vi "fpga_RefCounter.vi"(7 "reset":bool, 9 "input valid?":bool, 10 "Reference index":u8, 11 "NChan":u8) -> (1 "Reference channel input valid":bool, 3 "Multichannel enable":bool)   [LabVIEW 2011, in "NI_EP_Resample_FPGA.lvlib"]
uses:
  <vilib>/rvi/FXPMathLib/basic elements/FxpAddSub/XNode/nifxpmath_AddSub.xnode
  <vilib>/addons/Electrical Power/PQ/Resampling/NI_EP_Resample_FPGA.lvlib
  <vilib>/rvi/FXPMathLib/sim/FxpSim.dll
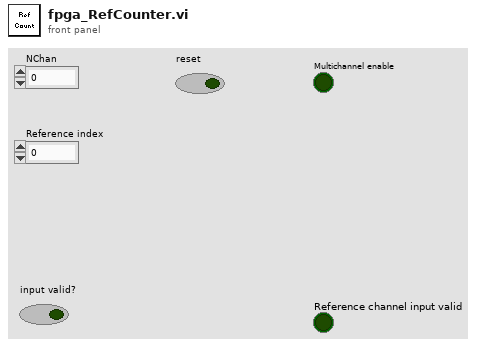
[diagram p1: front panel]
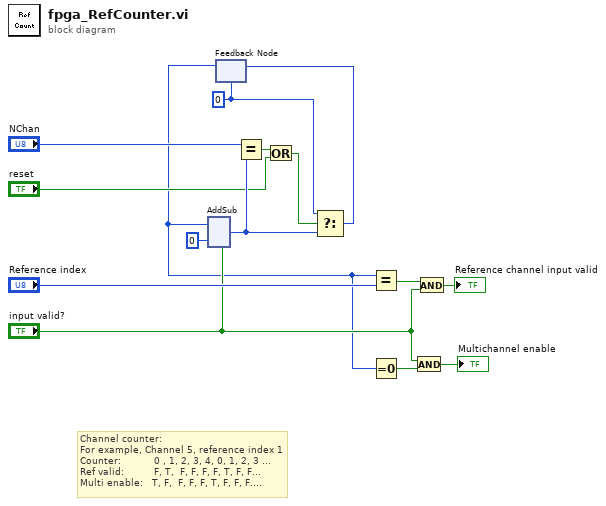
[diagram p0: block diagram]
diagram:
  w9 = u8 0 ("s")
  # "Channel counter:\nFor example, Channel 5, reference index 1\nCounter:           0 , 1, 2, 3, 4, 0, 1, 2, 3 ...\nRef valid:          F, T,  F, F, F, F, T, F, F...\nMulti enable:   T, F,  F, F, F, T, F, F, F...."
  n1 = feedback #1(w9) -> (w1:u8)
  n2 = xnode "AddSub"("x"=w1, "y"=u8 0, "carry-in"="input valid?") -> ("s"=w5:u8)  [unwired: 1 out]
  n3 = Equal?(x="NChan", y=w5) -> (x = y?=w4:bool)
  n4 = Or(x=w4, y="reset") -> (x .or. y?=w2:bool)
  n5 = Select(t=w9, s=w2, f=w5) -> (s? t:f=w8:u8)
  n6 = feedback-in #1(w8) -> ()
  n7 = Equal?(x=w1, y="Reference index") -> (x = y?=w14:bool)
  n8 = Equal To 0?(x=w1) -> (x = 0?=w12:bool)
  n9 = And(x="input valid?", y=w12) -> (x .and. y?=→"Multichannel enable":bool)
  n10 = And(x=w14, y="input valid?") -> (x .and. y?=→"Reference channel input valid":bool)
